vi "tsdb_unload_can_dbs.vi"(8 "错误输入（无错误）":errorcluster, 11 "path":path) -> (0 "错误输出":errorcluster, 2 "Return Type":i32, 3 "path out":path)   [LabVIEW 2014]
doc: "Function Introduction :\nUninstall all loaded DBC files\nCall location :\nThis function must be executed before or after the application is in a disconnected state (before executing tsapp_comnect)\nTsapp_disconnect). When the application is in a connected state, it cannot be deleted,\nLoad the database file.\ninput parameter :\nnothing\nReturn value :\n==0: Execution successful\nOther values: Query error code"
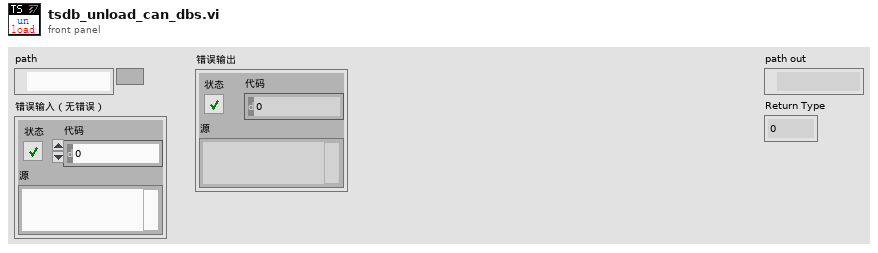
[diagram p1: front panel]
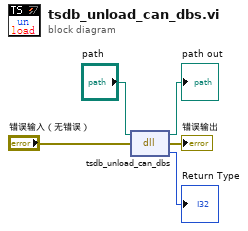
[diagram p0: block diagram]
diagram:
  n1 = dll-call lib="C:/Users/XYY/Desktop/LabView Demo/TSCAN_LB2018_V1.4_20220309/Config/TSMaster.dll" fn="tsdb_unload_can_dbs"(path in="path", error in="错误输入（无错误）") -> (path out=→"path out":path, error out=→"错误输出":errorcluster, "返回类型"=→"Return Type":i32)  [unwired: 1 in]
